vi "niFpgaButterflyTemp_4Pipe.vi"(0 "x_r":fxp<+/-,16,1>, 1 "mult output type":fxp<+/-,18,2>, 2 "bf bullet type":fxp<+/-,32,16> format="%.21g", 5 "x_i":fxp<+/-,16,1>, 7 "y_r":fxp<+/-,16,1>, 9 "y_i":fxp<+/-,16,1>, 12 "tf_r":fxp<+/-,16,1>, 13 "tf_i":fxp<+/-,16,1>, 14 "first stage":bool) -> (4 "x_out_r":fxp<+/-,16,1>, 6 "x_out_i":fxp<+/-,16,1>, 8 "y_out_r":fxp<+/-,16,1>, 10 "y_out_i":fxp<+/-,16,1>)   [LabVIEW 2017]
uses:
  <vilib>/rvi/FXPMathLib/FxpMul/XNode/nifxpmath_Multiplier.xnode
  <vilib>/rvi/FXPMathLib/sim/FxpSim.dll
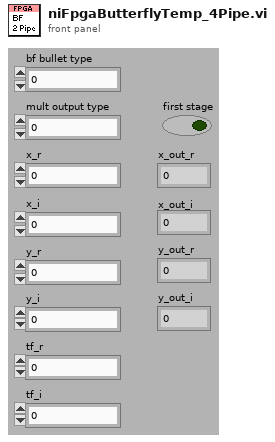
[diagram p1: front panel]
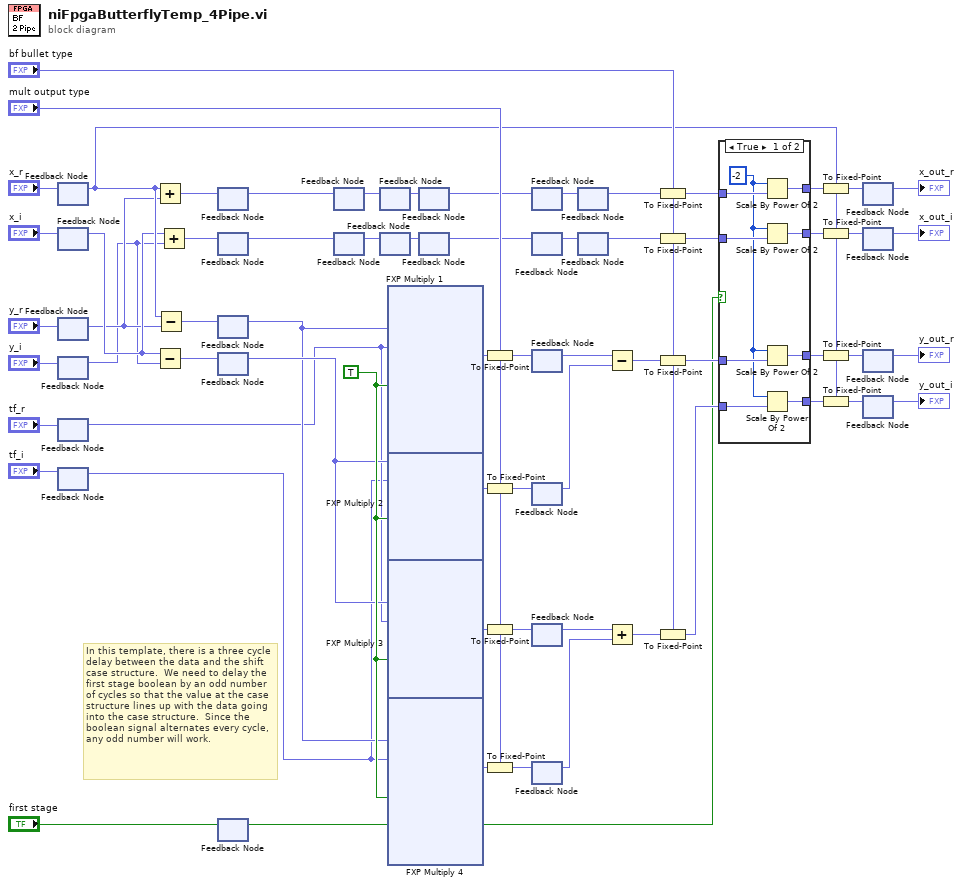
[diagram p0: block diagram]
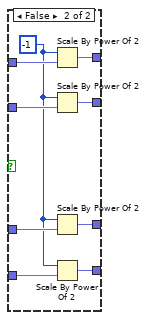
[diagram p2: hidden frame]
diagram:
  w56 = TRUE ("input valid")
  # "In this template, there is a three cycle delay between the data and the shift case structure.  We need to delay the first stage boolean by an odd number of cycles so that the value at the case structure lines up with the data going into the case structure.  Since the boolean signal alternates every cycle, any odd number will work."
  n1 = feedback-in #1("x_r") -> ()
  n2 = feedback #1() -> (w12:fxp<+/-,16,1>)  [unwired: 1 out]
  n3 = feedback-in #2("x_i") -> ()
  n4 = feedback #2() -> (w11:fxp<+/-,16,1>)  [unwired: 1 out]
  n5 = feedback-in #3("y_r") -> ()
  n6 = feedback #3() -> (w10:fxp<+/-,16,1>)  [unwired: 1 out]
  n7 = feedback-in #4("y_i") -> ()
  n8 = feedback #4() -> (w9:fxp<+/-,16,1>)  [unwired: 1 out]
  n9 = feedback-in #5("tf_r") -> ()
  n10 = feedback #5() -> (w8:fxp<+/-,16,1>)  [unwired: 1 out]
  n11 = feedback-in #6("tf_i") -> ()
  n12 = feedback #6() -> (w7:fxp<+/-,16,1>)  [unwired: 1 out]
  n13 = Add(x=w12, y=w10) -> (x+y=w53:fxp<+/-,17,2>)
  n14 = Subtract(x=w11, y=w9) -> (x-y=w64:fxp<+/-,17,2>)
  n15 = Subtract(x=w12, y=w10) -> (x-y=w65:fxp<+/-,17,2>)
  n16 = Add(x=w11, y=w9) -> (x+y=w36:fxp<+/-,17,2>)
  n17 = feedback-in #7(w53) -> ()
  n18 = feedback #7() -> (w40:fxp<+/-,17,2>)  [unwired: 1 out]
  n19 = feedback-in #8(w36) -> ()
  n20 = feedback #8() -> (w38:fxp<+/-,17,2>)  [unwired: 1 out]
  n21 = feedback-in #9(w65) -> ()
  n22 = feedback #9() -> (w34:fxp<+/-,17,2>)  [unwired: 1 out]
  n23 = feedback-in #10(w64) -> ()
  n24 = feedback #10() -> (w35:fxp<+/-,17,2>)  [unwired: 1 out]
  n25 = feedback-in #11("first stage") -> ()
  n26 = feedback #11() -> (w28:bool)  [unwired: 1 out]
  n27 = feedback-in #12(w40) -> ()
  n28 = feedback #12() -> (w39:fxp<+/-,17,2>)  [unwired: 1 out]
  n29 = feedback-in #13(w38) -> ()
  n30 = feedback #13() -> (w37:fxp<+/-,17,2>)  [unwired: 1 out]
  n31 = feedback-in #14(w39) -> ()
  n32 = feedback #14() -> (w23:fxp<+/-,17,2>)  [unwired: 1 out]
  n33 = feedback-in #15(w37) -> ()
  n34 = feedback #15() -> (w24:fxp<+/-,17,2>)  [unwired: 1 out]
  n35 = xnode "FXP Multiply 1"("x"=w34, "y"=w8, "input valid"=w56) -> ("x*y"=w29:fxp<+/-,33,3>)  [unwired: 1 in, 2 out]
  n36 = xnode "FXP Multiply 2"("x"=w35, "y"=w7, "input valid"=w56) -> ("x*y"=w50:fxp<+/-,33,3>)  [unwired: 1 in, 2 out]
  n37 = xnode "FXP Multiply 3"("x"=w35, "y"=w8, "input valid"=w56) -> ("x*y"=w51:fxp<+/-,33,3>)  [unwired: 1 in, 2 out]
  n38 = xnode "FXP Multiply 4"("x"=w34, "y"=w7, "input valid"=w56) -> ("x*y"=w52:fxp<+/-,33,3>)  [unwired: 1 in, 2 out]
  n39 = feedback-in #16(w23) -> ()
  n40 = feedback #16() -> (w6:fxp<+/-,17,2>)  [unwired: 1 out]
  n41 = feedback-in #17(w24) -> ()
  n42 = feedback #17() -> (w5:fxp<+/-,17,2>)  [unwired: 1 out]
  n43 = To Fixed-Point(fixed-point type="mult output type", number=w29) -> (fixed-point=w20:fxp<+/-,18,2>)
  n44 = To Fixed-Point(fixed-point type="mult output type", number=w50) -> (fixed-point=w19:fxp<+/-,18,2>)
  n45 = To Fixed-Point(fixed-point type="mult output type", number=w51) -> (fixed-point=w18:fxp<+/-,18,2>)
  n46 = To Fixed-Point(fixed-point type="mult output type", number=w52) -> (fixed-point=w17:fxp<+/-,18,2>)
  n47 = feedback-in #18(w6) -> ()
  n48 = feedback #18() -> (w25:fxp<+/-,17,2>)  [unwired: 1 out]
  n49 = feedback-in #19(w5) -> ()
  n50 = feedback #19() -> (w26:fxp<+/-,17,2>)  [unwired: 1 out]
  n51 = feedback-in #20(w20) -> ()
  n52 = feedback #20() -> (w13:fxp<+/-,18,2>)  [unwired: 1 out]
  n53 = feedback-in #21(w19) -> ()
  n54 = feedback #21() -> (w14:fxp<+/-,18,2>)  [unwired: 1 out]
  n55 = feedback-in #22(w18) -> ()
  n56 = feedback #22() -> (w15:fxp<+/-,18,2>)  [unwired: 1 out]
  n57 = feedback-in #23(w17) -> ()
  n58 = feedback #23() -> (w16:fxp<+/-,18,2>)  [unwired: 1 out]
  n59 = feedback-in #24(w25) -> ()
  n60 = feedback #24() -> (w22:fxp<+/-,17,2>)  [unwired: 1 out]
  n61 = feedback-in #25(w26) -> ()
  n62 = feedback #25() -> (w21:fxp<+/-,17,2>)  [unwired: 1 out]
  n63 = Subtract(x=w13, y=w14) -> (x-y=w45:fxp<+/-,19,3>)
  n64 = Add(x=w15, y=w16) -> (x+y=w47:fxp<+/-,19,3>)
  n65 = To Fixed-Point(fixed-point type="bf bullet type", number=w22) -> (fixed-point=w43:fxp<+/-,32,16>)
  n66 = To Fixed-Point(fixed-point type="bf bullet type", number=w21) -> (fixed-point=w42:fxp<+/-,32,16>)
  n67 = To Fixed-Point(fixed-point type="bf bullet type", number=w45) -> (fixed-point=w44:fxp<+/-,32,16>)
  n68 = To Fixed-Point(fixed-point type="bf bullet type", number=w47) -> (fixed-point=w46:fxp<+/-,32,16>)
  n69 = case shown="True" w28 {
    tunnel: [w74 w83] -> w60
    tunnel: [w73 w82] -> w59
    tunnel: [w72 w81] -> w58
    tunnel: [w71 w80] -> w57
    tunnel: w46 -> [w70 w79]
    tunnel: w44 -> [w69 w78]
    tunnel: w43 -> [w68 w77]
    tunnel: w42 -> [w67 w76]
    frame True {
      w66 = -2 ("n")
      n70 = Scale By Power Of 2(n=w66, x=w68) -> (x*2^n=w74:fxp<+/-,32,16>)
      n71 = Scale By Power Of 2(n=w66, x=w67) -> (x*2^n=w73:fxp<+/-,32,16>)
      n72 = Scale By Power Of 2(n=w66, x=w69) -> (x*2^n=w72:fxp<+/-,32,16>)
      n73 = Scale By Power Of 2(n=w66, x=w70) -> (x*2^n=w71:fxp<+/-,32,16>)
    }
    frame False {
      w75 = -1 ("n")
      n74 = Scale By Power Of 2(n=w75, x=w77) -> (x*2^n=w83:fxp<+/-,32,16>)
      n75 = Scale By Power Of 2(n=w75, x=w76) -> (x*2^n=w82:fxp<+/-,32,16>)
      n76 = Scale By Power Of 2(n=w75, x=w78) -> (x*2^n=w81:fxp<+/-,32,16>)
      n77 = Scale By Power Of 2(n=w75, x=w79) -> (x*2^n=w80:fxp<+/-,32,16>)
    }
  }
  n78 = To Fixed-Point(fixed-point type=w12, number=w60) -> (fixed-point=w32:fxp<+/-,16,1>)
  n79 = To Fixed-Point(fixed-point type=w12, number=w59) -> (fixed-point=w33:fxp<+/-,16,1>)
  n80 = To Fixed-Point(fixed-point type=w12, number=w58) -> (fixed-point=w31:fxp<+/-,16,1>)
  n81 = To Fixed-Point(fixed-point type=w12, number=w57) -> (fixed-point=w30:fxp<+/-,16,1>)
  n82 = feedback-in #26(w32) -> ()
  n83 = feedback #26() -> (→"x_out_r":fxp<+/-,16,1>)  [unwired: 1 out]
  n84 = feedback-in #27(w33) -> ()
  n85 = feedback #27() -> (→"x_out_i":fxp<+/-,16,1>)  [unwired: 1 out]
  n86 = feedback-in #28(w31) -> ()
  n87 = feedback #28() -> (→"y_out_r":fxp<+/-,16,1>)  [unwired: 1 out]
  n88 = feedback-in #29(w30) -> ()
  n89 = feedback #29() -> (→"y_out_i":fxp<+/-,16,1>)  [unwired: 1 out]
